vi "getParaTypeNum.vi"(6 "testEnd":bool, 7 "paraSN":i32, 8 "lastTimeLoopParaExist?":bool, 9 "lastTimeLoopParaEndNumArr":i32[](array[numeric]), 10 "lastTimeLoopParaStartNumArr":i32[](array[numeric]), 11 "parameter":string) -> (0 "thisTimeLoopParaExist?":bool, 1 "thisTimeLoopParaEndNumArr":i32[](array[numeric]), 2 "thisTimeLoopParaStartNumArr":i32[](array[numeric]))   [LabVIEW 2010]
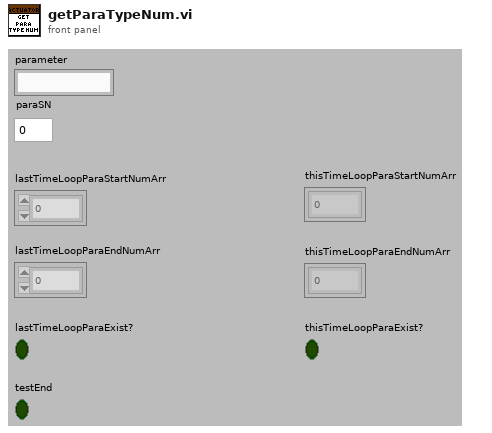
[diagram p1: front panel]
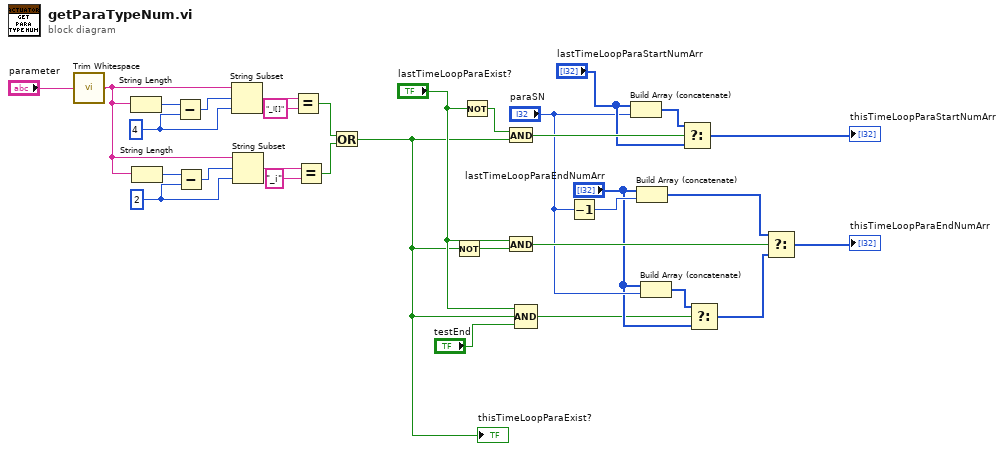
[diagram p0: block diagram]
diagram:
  w28 = 2 ("y")
  w30 = 4 ("y")
  n1 = call <vilib>:"Trim Whitespace.vi"("string"="parameter") -> ("trimmed string"=w25:string)  [unwired: 1 in]
  n2 = String Length(string=w25) -> (length=w32:i32)
  n3 = String Length(string=w25) -> (length=w26:i32)
  n4 = Subtract(x=w32, y=w30) -> (x-y=w31:i32)
  n5 = Subtract(x=w26, y=w28) -> (x-y=w27:i32)
  n6 = String Subset(string=w25, offset (0)=w31, length (rest)=w30) -> (substring=w24:string)
  n7 = String Subset(string=w25, offset (0)=w27, length (rest)=w28) -> (substring=w22:string)
  n8 = Equal?(x=w24, y="_i[]") -> (x = y?=w20:bool)
  n9 = Equal?(x=w22, y="_i") -> (x = y?=w19:bool)
  n10 = Or(x=w20, y=w19) -> (x .or. y?=w3:bool)
  "thisTimeLoopParaExist?" <- w3
  n11 = Not(x=w3) -> (.not. x?=w13:bool)
  n12 = Not(x="lastTimeLoopParaExist?") -> (.not. x?=w18:bool)
  n13 = And(x=w18, y=w3) -> (x .and. y?=w17:bool)
  n14 = And(x="lastTimeLoopParaExist?", y=w13) -> (x .and. y?=w12:bool)
  n15 = Compound Arithmetic op=AND("lastTimeLoopParaExist?", w3, "testEnd") -> (w1:bool)
  n16 = Decrement(x="paraSN") -> (x-1=w11:i32)
  n17 = Build Array (concatenate)("lastTimeLoopParaStartNumArr", "paraSN") -> (w16:i32[])
  n18 = Build Array (concatenate)("lastTimeLoopParaEndNumArr", w11) -> (w10:i32[])
  n19 = Build Array (concatenate)("lastTimeLoopParaEndNumArr", "paraSN") -> (w7:i32[])
  n20 = Select(t=w16, s=w17, f="lastTimeLoopParaStartNumArr") -> (s? t:f=→"thisTimeLoopParaStartNumArr":i32[])
  n21 = Select(t=w7, s=w1, f="lastTimeLoopParaEndNumArr") -> (s? t:f=w5:i32[])
  n22 = Select(t=w10, s=w12, f=w5) -> (s? t:f=→"thisTimeLoopParaEndNumArr":i32[])
